vi "_main_abstractFactory.vi"() -> ()   [LabVIEW 2023, in "AbstractFactory.lvlib"]
uses:
  AbstractFactory.lvlib
  LegacyOvenFactory/LegacyOvenFactory.lvclass
  ModernOvenFactory/ModernOvenFactory.lvclass
  OvenController/OvenController.lvclass
panel:
  in  "ovenSelection":enum16{"LegacyOven", "ModernOven"}(ring)
  out "currentTemperature[°C]":i32
  in  "desiredTemperature[°C]":i32=85
  # "ABSTRACT FACTORY"
  # "INSTRUCTIONS:\n- Set the desired oven type: legacy or moden oven.\n- Set the desired temperature.\n- Run the code.\n- See comments in the block diagram"
  # "Select and run VI"
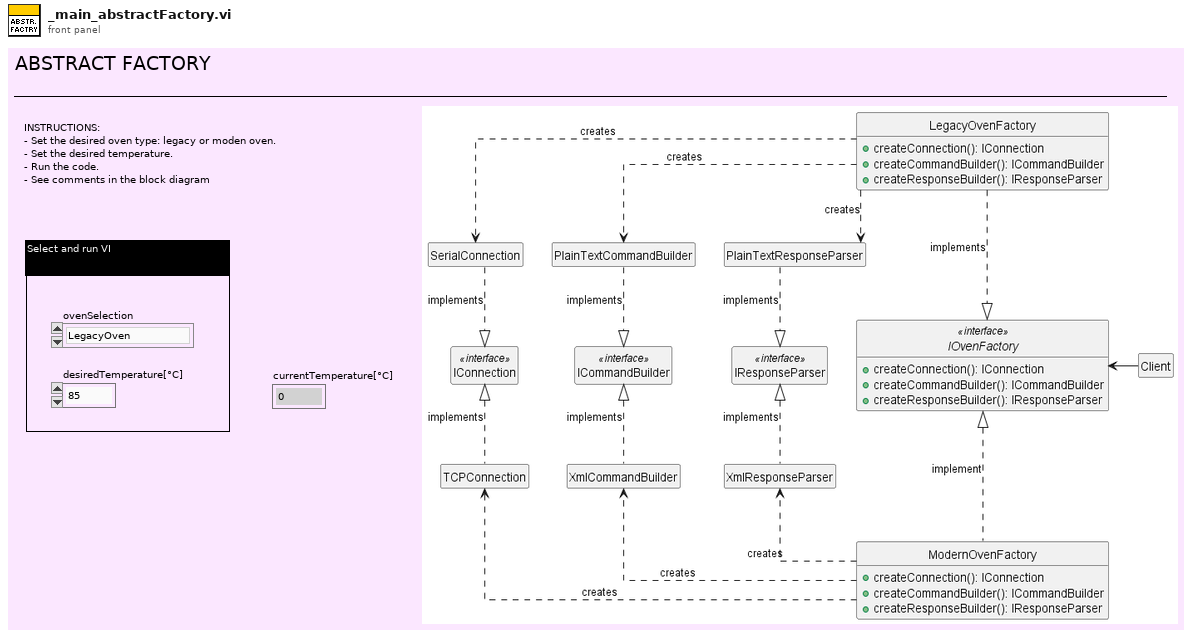
[diagram p1: front panel]
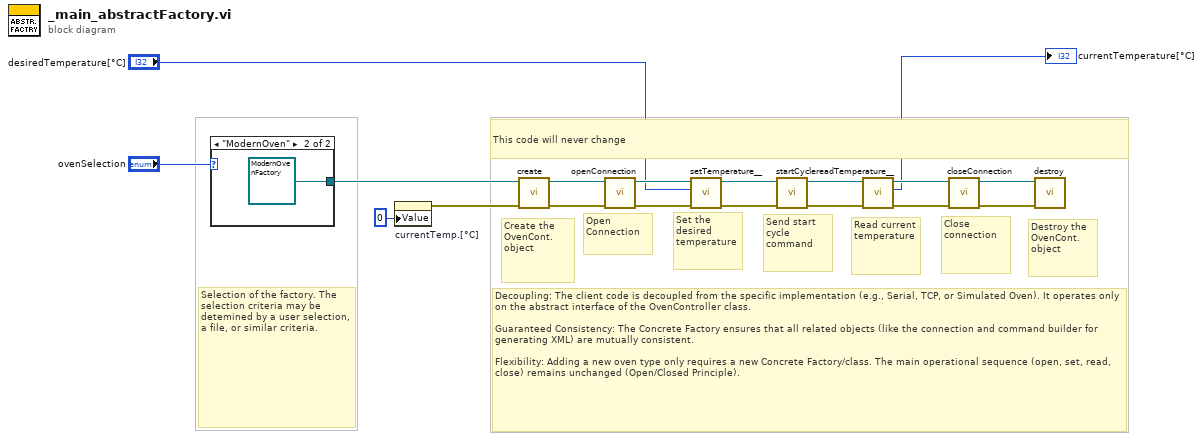
[diagram p0: block diagram]
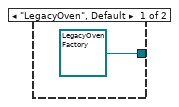
[diagram p2: hidden frame]
diagram:
  # "This code will never change"
  # "Selection of the factory. The selection criteria may be detemined by a user selection, a file, or similar criteria."
  # "Decoupling: The client code is decoupled from the specific implementation (e.g., Serial, TCP, or Simulated Oven). It operates only on the abstract interface of the OvenController class.\n\nGuaranteed Consistency: The Concrete Factory ensures that all related objects (like the connection and command builder for generating XML) are mutually consistent.\n\nFlexibility: Adding a new oven type only requires a new Concrete Factory/class. The main operational sequence (open, set, read, close) remains unchanged (Open/Closed Principle)."
  # "Destroy the OvenCont. object"
  # "Create the OvenCont. object"
  # "Close connection"
  # "Read current temperature"
  # "Send start cycle command"
  # "Set the desired temperature"
  # "Open Connection"
  n1 = case shown="\"ModernOven\"" "ovenSelection" {
    tunnel: [refnum<class "LegacyOvenFactory.lvclass"> refnum ("AbstractFactory.lvlib:LegacyOvenFactory.lvclass") refnum<class "ModernOvenFactory.lvclass"> refnum ("AbstractFactory.lvlib:ModernOvenFactory.lvclass")] -> w3
    frame "LegacyOven", Default {
    }
    frame "ModernOven" {
    }
  }
  n2 = property on="currentTemp.[°C]" class="DigNum (strict)"("Value"=0 ("currentTemperature[°C]")) -> (error out=w1:errorcluster)  [unwired: 2 in, 1 out]
  n3 = call "create.vi"("error in (no error)"=w1, "IOvenFactory"=w3) -> ("error out"=w18:errorcluster, "OvenController out"=w13:refnum<class "OvenController.lvclass">)  [unwired: 8 in]
  n4 = call "openConnection.vi"("error in (no error)"=w18, "OvenController in"=w13) -> ("error out"=w17:errorcluster, "OvenController out"=w12:refnum<class "OvenController.lvclass">)  [unwired: 8 in]
  n5 = call "setTemperature__.vi"("error in (no error)"=w17, "temperature[°C]"="desiredTemperature[°C]", "OvenController in"=w12) -> ("error out"=w16:errorcluster, "OvenController out"=w11:refnum<class "OvenController.lvclass">)  [unwired: 7 in]
  n6 = call "startCycle.vi"("error in (no error)"=w16, "OvenController in"=w11) -> ("error out"=w15:errorcluster, "OvenController out"=w10:refnum<class "OvenController.lvclass">)  [unwired: 8 in]
  n7 = call "readTemperature__.vi"("error in (no error)"=w15, "OvenController in"=w10) -> ("error out"=w14:errorcluster, "temperature[°C]"=→"currentTemperature[°C]":i32, "OvenController out"=w9:refnum<class "OvenController.lvclass">)  [unwired: 7 in]
  n8 = call "closeConnection.vi"("error in (no error)"=w14, "OvenController in"=w9) -> ("error out"=w6:errorcluster, "OvenController out"=w5:refnum<class "OvenController.lvclass">)  [unwired: 8 in]
  n9 = call "destroy.vi"("error in (no error)"=w6, "OvenController in"=w5) -> ()  [unwired: 9 in, 1 out]
